vi "Set Shutters.vi"(0 "typ":i32, 1 "exttype":i32, 2 "dummy1":i32, 5 "mode":i32, 7 "closingtime":i32, 9 "openingtime":i32, 11 "error in (no error)":errorcluster, 12 "extmode":i32, 13 "dummy2":i32) -> (4 "function return":u32, 15 "error out":errorcluster)   [LabVIEW 2014, in "atmcd32d.lvlib"]
doc: "unsigned int WINAPI SetShutters(int typ, int mode, int closingtime, int openingtime, int exttype, int extmode, int dummy1, int dummy2);"
uses:
  atmcd32d.lvlib
  atmcd32d.dll
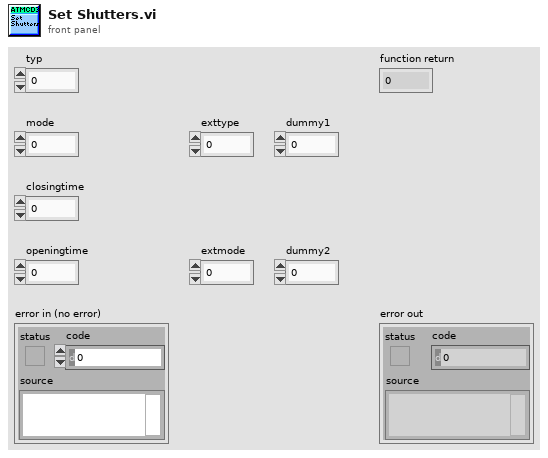
[diagram p1: front panel]
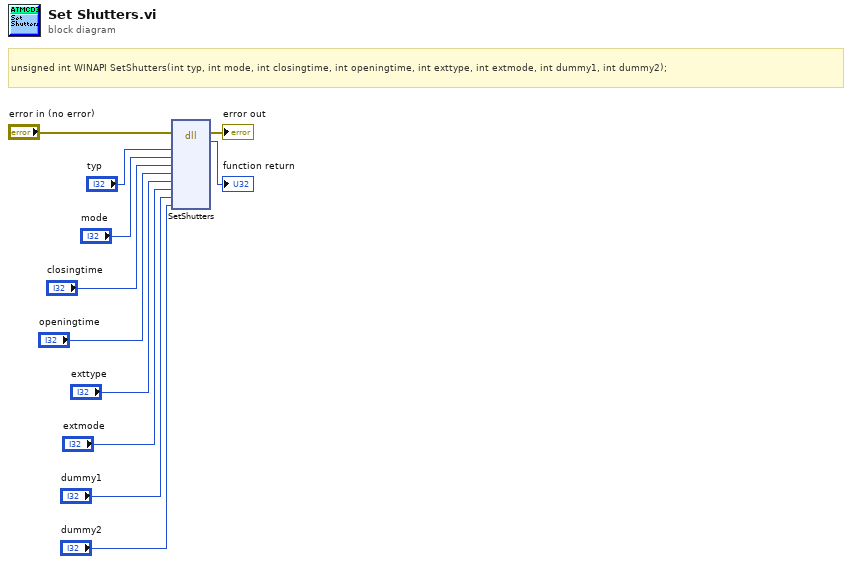
[diagram p0: block diagram]
diagram:
  # "unsigned int WINAPI SetShutters(int typ, int mode, int closingtime, int openingtime, int exttype, int extmode, int dummy1, int dummy2);"
  n1 = dll-call lib="C:/Users/Bakir/Documents/Lambda2-Testing/lib/Andorlib/atmcd32d.*" fn="SetShutters"(error in="error in (no error)", "typ"="typ", "mode"="mode", "closingtime"="closingtime", "openingtime"="openingtime", "exttype"="exttype", "extmode"="extmode", "dummy1"="dummy1", "dummy2"="dummy2") -> (error out=→"error out":errorcluster, →"function return":u32)  [unwired: 10 in, 1 out]
